vi "Get Product Number.vi"(8 "error in (no error)":errorcluster caption="entrée d'erreur (pas d'erreur)", 11 "Creation_SN_Nodon en entrée":refnum<class "Creation_SN_Nodon.lvclass">) -> (0 "error out":errorcluster caption="sortie d'erreur", 2 "Product Number":string="STPH", 3 "Creation_SN_Nodon en sortie":refnum<class "Creation_SN_Nodon.lvclass">)   [LabVIEW 2020, in "Library Instrument & Equipement.lvlib" / "Library Creation_SN.lvlib" / "Creation_SN_Nodon.lvclass"]
uses:
  Creation_SN_Nodon.lvclass
  Creation_SN_Nodon.lvclass/Creation_SN_Nodon.ctl
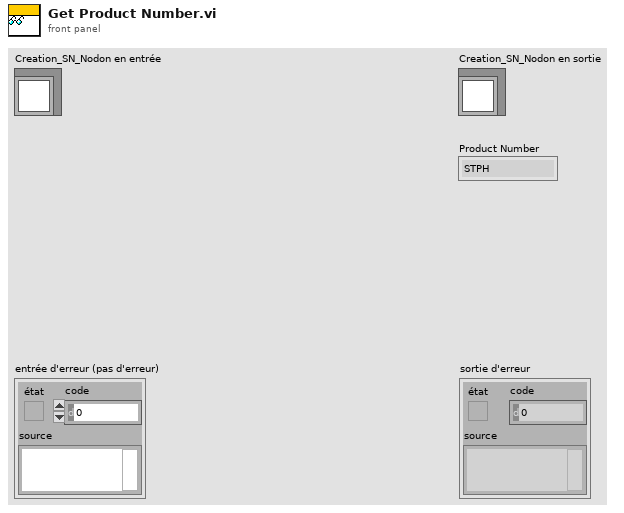
[diagram p1: front panel]
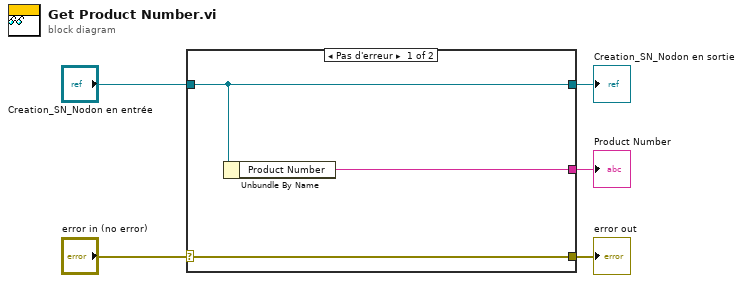
[diagram p0: block diagram]
diagram:
  n1 = case shown="Pas d'erreur" "error in (no error)" {
    selector: "error in (no error)" -> [w8 w9]
    tunnel: [w8 w9] -> w4
    tunnel: [w7 w10] -> w2
    tunnel: "Creation_SN_Nodon en entrée" -> [w7 w10]
    tunnel: [w6 _] -> w1
    frame No Error {
      n2 = Unbundle By Name(w7) -> ("Product Number"=w6:string)
    }
    frame Error {
    }
  }
  "error out" <- w4
  "Creation_SN_Nodon en sortie" <- w2
  "Product Number" <- w1
